vi "yearly breakdown query.vi"(6 "Year":string, 8 "error in":errorcluster, 9 "Shift":string, 10 "Station":string, 11 "Refnum in":T1) -> (0 "error out":errorcluster, 1 "Count":string[][](array[string]), 2 "Duration":string[][](array[string]), 3 "connection reference out":T1)   [LabVIEW 2017]
uses:
  <vilib>/addons/database/Connection.llb/Conn ObjectReference.ctl
  <vilib>/addons/database/NI_Database_API.lvlib
panel:
  in  "Month":string(combo)
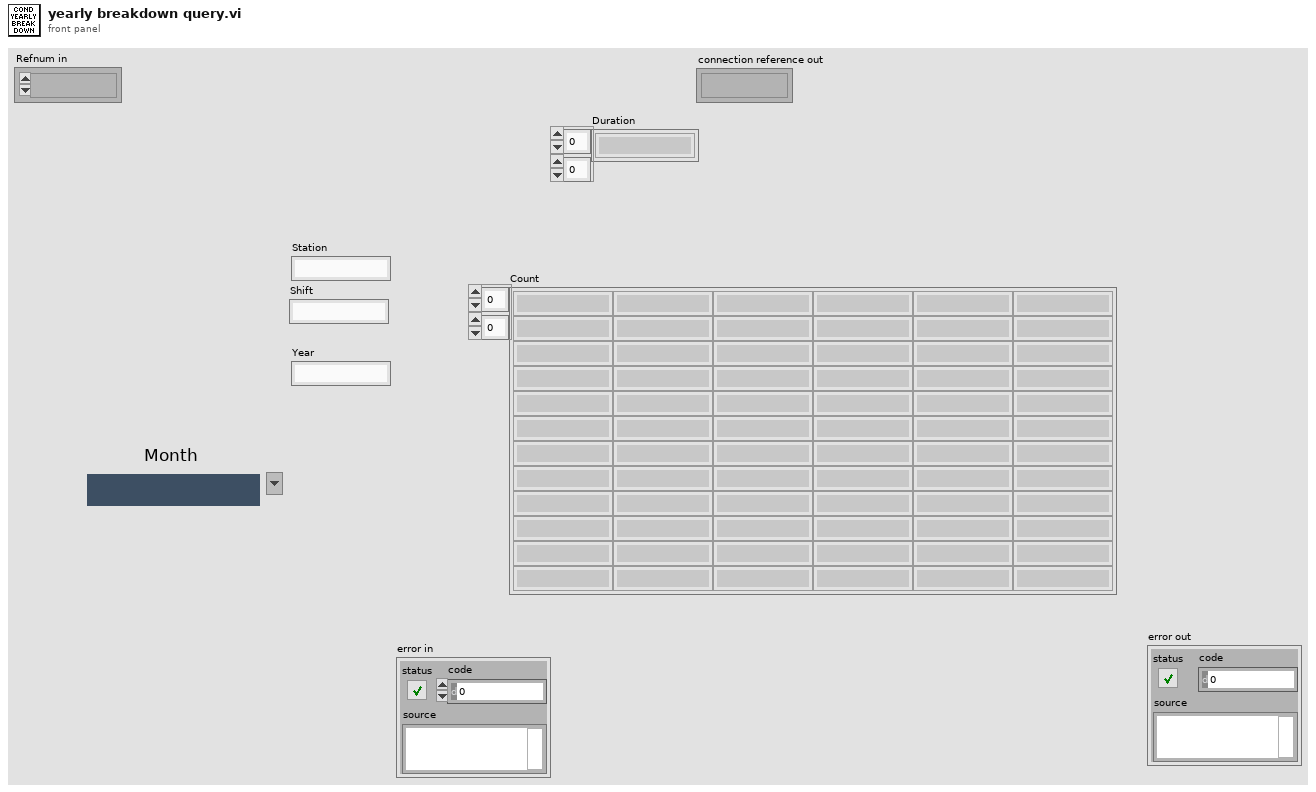
[diagram p1: front panel]
types:
  T1 = typedef "NI_Database_API.lvlib/Conn ObjectReference.ctl" = refnum<k1>
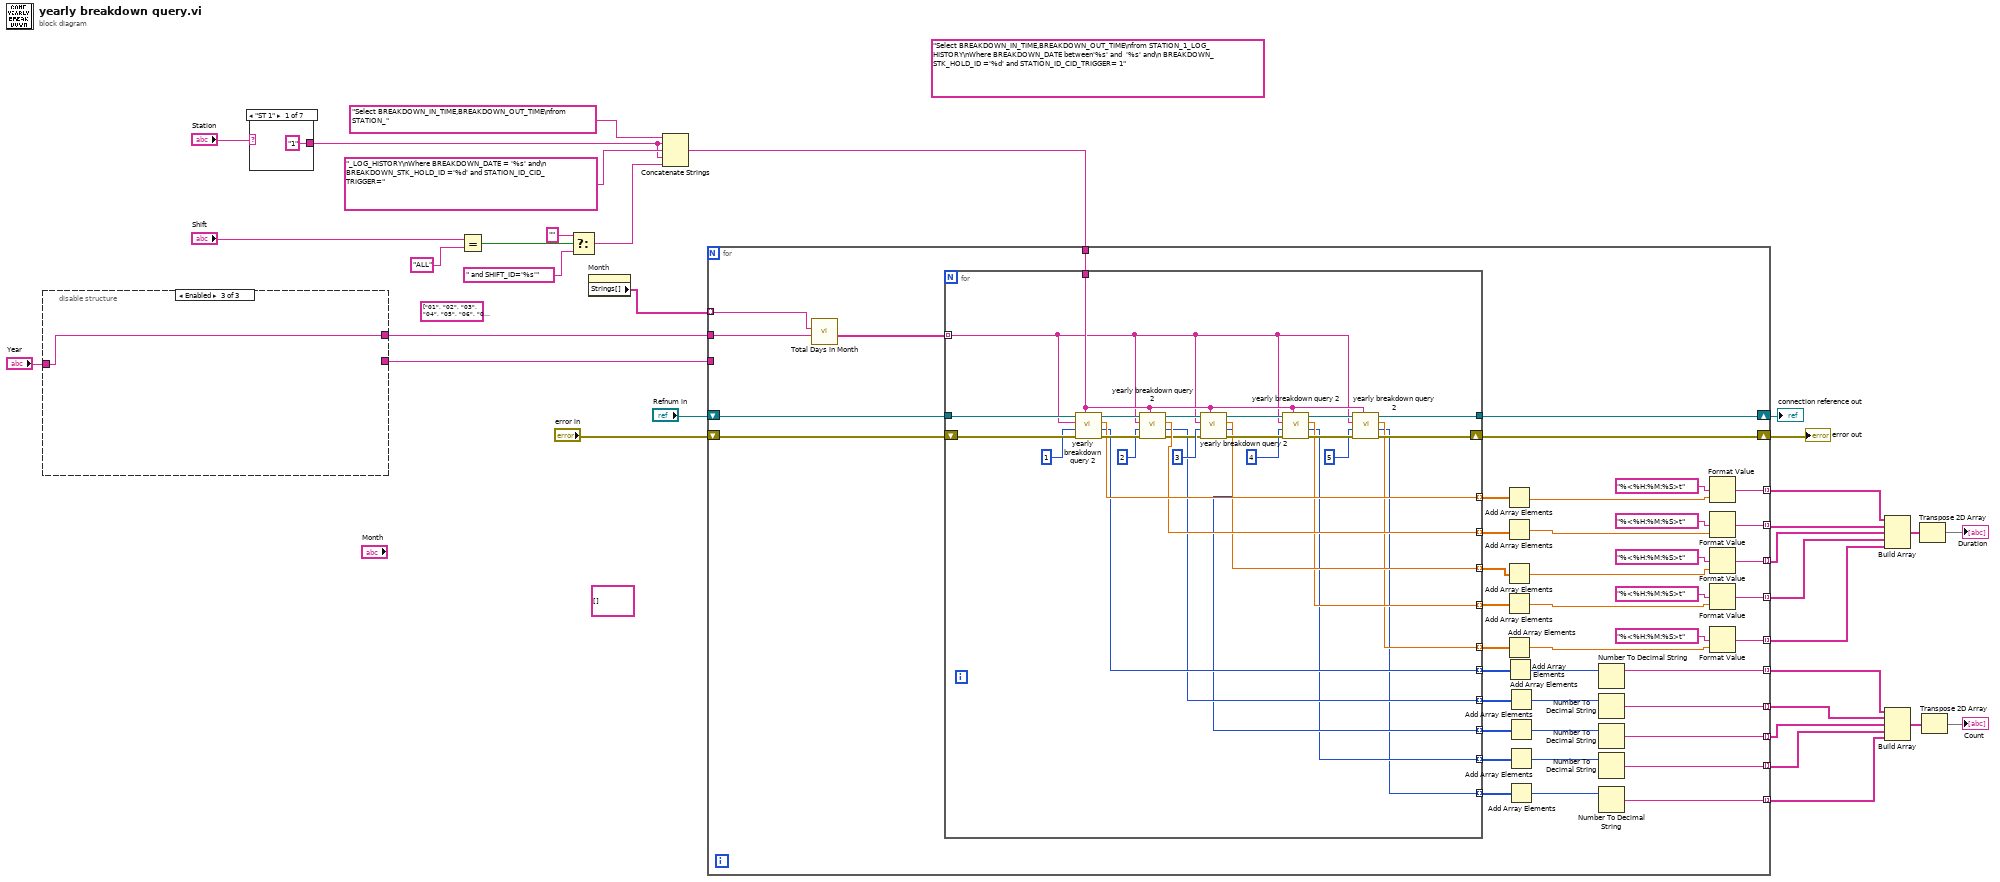
[diagram p0: block diagram]
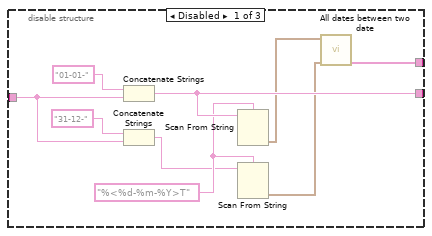
[diagram p2: hidden frame]
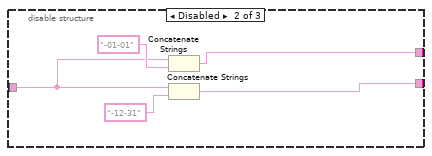
[diagram p3: hidden frame]
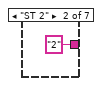
[diagram p4: hidden frame]
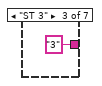
[diagram p5: hidden frame]
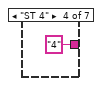
[diagram p6: hidden frame]
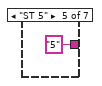
[diagram p7: hidden frame]
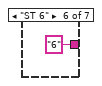
[diagram p8: hidden frame]
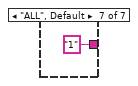
[diagram p9: hidden frame]
diagram:
  (unwired) string[] ["01", "02", "03", "04", "05", "06", "07", "08", "09", "10", "11", "12"]
  (unwired) string[][] [] ("Output Array")
  (unwired) "Select BREAKDOWN_IN_TIME,BREAKDOWN_OUT_TIME\nfrom STATION_1_LOG_HISTORY\nWhere BREAKDOWN_DATE between'%s' and  '%s' and\n BREAKDOWN_STK_HOLD_ID ='%d' and STATION_ID_CID_TRIGGER= 1"
  n1 = disable-structure shown="Enabled" {
    disable-tunnel: "Year" -> [w40 w45 w48]
    disable-tunnel: [w39 w43 _] -> w21
    disable-tunnel: [w34 w44 w48] -> w20
    frame Disabled {
      w38 = "%<%d-%m-%Y>T" ("format string")
      n2 = Concatenate Strings("01-01-" ("string"), w40) -> (w39:string)
      n3 = Concatenate Strings("31-12-" ("string"), w40) -> (w37:string)
      n4 = Scan From String(format string=w38, input string=w39) -> (output 1=w36:timestamp)  [unwired: 3 in, 3 out]
      n5 = Scan From String(format string=w38, input string=w37) -> (output 1=w35:timestamp)  [unwired: 3 in, 3 out]
      n6 = call "All dates between two date.vi"("To Date"=w35, "From Date"=w36) -> ("All Days (String)"=w34:string[])  [unwired: 8 in, 1 out]
    }
    frame Disabled {
      n7 = Concatenate Strings(w45, "-01-01" ("string")) -> (w44:string)
      n8 = Concatenate Strings(w45, "-12-31" ("string")) -> (w43:string)
    }
    frame Enabled {
    }
  }
  n9 = case shown="\"ST 1\"" "Station" {
    tunnel: ["1" "2" "3" "4" "5" "6" "1"] -> w27
    frame "ST 1" {
    }
    frame "ST 2" {
    }
    frame "ST 3" {
    }
    frame "ST 4" {
    }
    frame "ST 5" {
    }
    frame "ST 6" {
    }
    frame "ALL", Default {
    }
  }
  n10 = Equal?(x="Shift", y="ALL" ("condition")) -> (x = y?=w30:bool)
  n11 = Select(t="", s=w30, f=" and SHIFT_ID='%s'" ("condition")) -> (s? t:f=w26:string)
  n12 = property on="Month" class="CmbBox"() -> ("Strings[]"=w19:string[])  [unwired: 2 in, 2 out]
  n13 = Concatenate Strings("Select BREAKDOWN_IN_TIME,BREAKDOWN_OUT_TIME\nfrom STATION_" ("string"), w27, "_LOG_HISTORY\nWhere BREAKDOWN_DATE = '%s' and\n BREAKDOWN_STK_HOLD_ID ='%d' and STATION_ID_CID_TRIGGER=" ("string"), w27, w26) -> (w25:string)
  n14 = for {
    tunnel: w25 -> [w94]
    tunnel: w21 -> [_]
    tunnel: w20 -> [w92]
    shift-right: [w95] -> w4
    shift-left: "Refnum in" -> [w98]
    shift-right: [w96] -> w3
    shift-left: "error in" -> [w97]
    tunnel: w19 -> [w93] mode=indexing
    tunnel: [w75] -> w18 mode=indexing
    tunnel: [w74] -> w17 mode=indexing
    tunnel: [w73] -> w16 mode=indexing
    tunnel: [w72] -> w15 mode=indexing
    tunnel: [w71] -> w14 mode=indexing
    tunnel: [w64] -> w11 mode=indexing
    tunnel: [w59] -> w10 mode=indexing
    tunnel: [w58] -> w9 mode=indexing
    tunnel: [w57] -> w8 mode=indexing
    tunnel: [w56] -> w7 mode=indexing
    n15 = call "Total Days in Month.vi"("Year"=w92, "Month"=w93) -> ("All Days"=w91:string[])  [unwired: 8 in, 1 out]
    n16 = for {
      tunnel: w98 -> [w127]
      tunnel: [w119] -> w95
      tunnel: w94 -> [w116]
      shift-right: [w117] -> w96
      shift-left: w97 -> [w126]
      tunnel: w91 -> [w110] mode=indexing
      tunnel: [w109] -> w85 mode=indexing
      tunnel: [w108] -> w83 mode=indexing
      tunnel: [w107] -> w81 mode=indexing
      tunnel: [w106] -> w79 mode=indexing
      tunnel: [w105] -> w77 mode=indexing
      tunnel: [w103] -> w70 mode=indexing
      tunnel: [w102] -> w69 mode=indexing
      tunnel: [w101] -> w68 mode=indexing
      tunnel: [w100] -> w66 mode=indexing
      tunnel: [w99] -> w67 mode=indexing
      n17 = call "yearly breakdown query 2.vi"("String 2"=w116, "error in (no error)"=w126, 9:1, "String"=w110, "Refnum in"=w127) -> ("error out"=w118:errorcluster, "Count"=w103:i32, "sum"=w109:dbl, "Refnum out"=w120:T1)  [unwired: 3 in]
      n18 = call "yearly breakdown query 2.vi"("String 2"=w116, "error in (no error)"=w118, 9:2, "String"=w110, "Refnum in"=w120) -> ("error out"=w104:errorcluster, "Count"=w102:i32, "sum"=w108:dbl, "Refnum out"=w125:T1)  [unwired: 3 in]
      n19 = call "yearly breakdown query 2.vi"("String 2"=w116, "error in (no error)"=w104, 9:3, "String"=w110, "Refnum in"=w125) -> ("error out"=w122:errorcluster, "Count"=w101:i32, "sum"=w107:dbl, "Refnum out"=w121:T1)  [unwired: 3 in]
      n20 = call "yearly breakdown query 2.vi"("String 2"=w116, "error in (no error)"=w122, 9:4, "String"=w110, "Refnum in"=w121) -> ("error out"=w124:errorcluster, "Count"=w100:i32, "sum"=w106:dbl, "Refnum out"=w123:T1)  [unwired: 3 in]
      n21 = call "yearly breakdown query 2.vi"("String 2"=w116, "error in (no error)"=w124, 9:5, "String"=w110, "Refnum in"=w123) -> ("error out"=w117:errorcluster, "Count"=w99:i32, "sum"=w105:dbl, "Refnum out"=w119:T1)  [unwired: 3 in]
    }
    n22 = Add Array Elements(numeric array=w85) -> (sum=w84:dbl)
    n23 = Add Array Elements(numeric array=w83) -> (sum=w82:dbl)
    n24 = Add Array Elements(numeric array=w81) -> (sum=w80:dbl)
    n25 = Add Array Elements(numeric array=w79) -> (sum=w78:dbl)
    n26 = Add Array Elements(numeric array=w77) -> (sum=w76:dbl)
    n27 = Add Array Elements(numeric array=w70) -> (sum=w65:i32)
    n28 = Add Array Elements(numeric array=w69) -> (sum=w60:i32)
    n29 = Add Array Elements(numeric array=w68) -> (sum=w61:i32)
    n30 = Add Array Elements(numeric array=w66) -> (sum=w62:i32)
    n31 = Add Array Elements(numeric array=w67) -> (sum=w63:i32)
    n32 = Number To Decimal String(number=w65) -> (decimal integer string=w64:string)  [unwired: 1 in]
    n33 = Number To Decimal String(number=w60) -> (decimal integer string=w59:string)  [unwired: 1 in]
    n34 = Number To Decimal String(number=w61) -> (decimal integer string=w58:string)  [unwired: 1 in]
    n35 = Number To Decimal String(number=w62) -> (decimal integer string=w57:string)  [unwired: 1 in]
    n36 = Number To Decimal String(number=w63) -> (decimal integer string=w56:string)  [unwired: 1 in]
    n37 = Format Value(format string="%<%H:%M:%S>t", value (0)=w84) -> (output string=w75:string)  [unwired: 1 in]
    n38 = Format Value(format string="%<%H:%M:%S>t", value (0)=w82) -> (output string=w74:string)  [unwired: 1 in]
    n39 = Format Value(format string="%<%H:%M:%S>t", value (0)=w80) -> (output string=w73:string)  [unwired: 1 in]
    n40 = Format Value(format string="%<%H:%M:%S>t", value (0)=w78) -> (output string=w72:string)  [unwired: 1 in]
    n41 = Format Value(format string="%<%H:%M:%S>t", value (0)=w76) -> (output string=w71:string)  [unwired: 1 in]
  }
  "connection reference out" <- w4
  "error out" <- w3
  n42 = Build Array(w18, w17, w16, w15, w14) -> (w13:string[][])
  n43 = Build Array(w11, w10, w9, w8, w7) -> (w12:string[][])
  n44 = Transpose 2D Array(2D array=w13) -> (transposed array=→"Duration":string[][])
  n45 = Transpose 2D Array(2D array=w12) -> (transposed array=→"Count":string[][])
